vi "ELOG_AggregationPeriod_Set.vi"(8 "error in (no error)":errorcluster, 10 "Period Duration (s)":dbl format="%#_13g", 11 "OXY_SCPI Reseource In":refnum<visa-resource-name>) -> (0 "error out":errorcluster, 1 "communication_data":T1, 3 "OXY_SCPI Reseource Out":refnum<visa-resource-name>)   [LabVIEW 2018, in "OXYGEN.lvlib"]
doc: "Sets the duration (in seconds) of the data aggregation time of statistics from source channels"
uses:
  OXYGEN.lvlib
  TypeDefs/Cluster_RawCommData.ctl
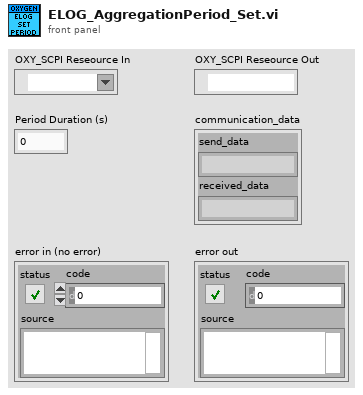
[diagram p1: front panel]
types:
  T1 = typedef "OXYGEN.lvlib/Cluster_RawCommData.ctl" = cluster{"send_data":string, "received_data":string}
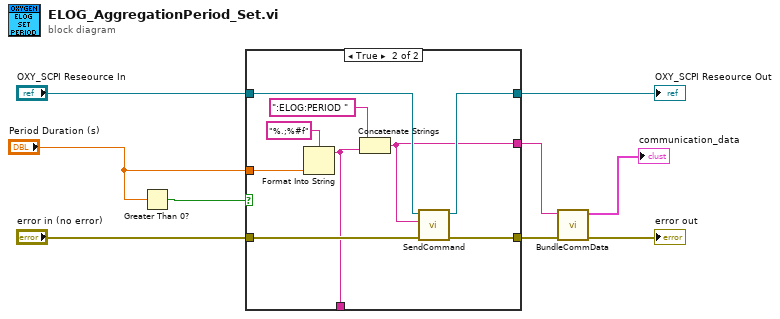
[diagram p0: block diagram]
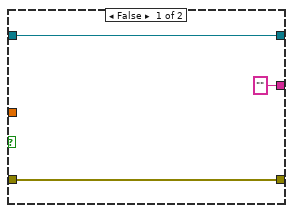
[diagram p2: hidden frame]
diagram:
  n1 = Greater Than 0?(x="Period Duration (s)") -> (x > 0?=w1:bool)
  n2 = case shown="True" w1 {
    tunnel: "error in (no error)" -> [w10 w20]
    tunnel: [w10 w19] -> w3
    tunnel: [w12 w18] -> w8
    tunnel: "OXY_SCPI Reseource In" -> [w12 w17]
    tunnel: "Period Duration (s)" -> [_ w15]
    tunnel: ["" w16] -> w6
    tunnel: [_ w13] -> _
    frame False {
    }
    frame True {
      n3 = Format Into String(format string="%.;%#f", w15) -> (resulting string=w13:string)  [unwired: 2 in, 1 out]
      n4 = Concatenate Strings(":ELOG:PERIOD " ("string"), w13) -> (w16:string)
      n5 = call "SendCommand.vi"("error in (no error)"=w20, "String to Send"=w16, "OXY_SCPI Reseource In"=w17) -> ("error out"=w19:errorcluster, "OXY_SCPI Reseource Out"=w18:refnum<visa-resource-name>)  [unwired: 7 in]
    }
  }
  "OXY_SCPI Reseource Out" <- w8
  n6 = call "BundleCommData.vi"("error in (no error)"=w3, "send_data"=w6) -> ("error out"=→"error out":errorcluster, "communication_data"=→"communication_data":T1)  [unwired: 8 in]
